vi "Reset.vi"(8 "error in (no error)":errorcluster, 9 "Mask":u64=16 format="x%x (b%b)", 10 "Set decimation":bool=TRUE, 11 "RP Instrument in":refnum<class "RP Instrument.lvclass">) -> (0 "error out":errorcluster, 3 "RP Instrument out":refnum<class "RP Instrument.lvclass">)   [LabVIEW 2024, in "RP Instrument.lvclass"]
uses:
  RP Instrument.lvclass
  RP Command.ctl
  RP Instrument.lvclass/RP Instrument.ctl
  RP Communicator/RP Communicator.lvclass
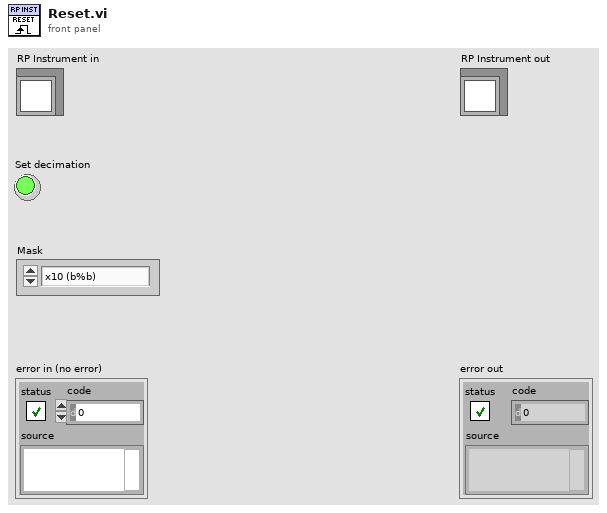
[diagram p1: front panel]
types:
  T1 = typedef "RP Command.ctl" = enum16{"Reset", "Read IDN", "Stop server", "Get status", "Get temperature", "Connect client", "Arm", "Software trigger", "Get whole buffer", "Get chunk", "System call", "Get config", "Set config", "Recieve data", "Recieve Calibartion", "Transmit data"}
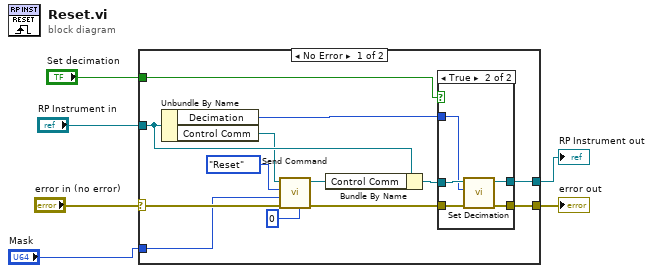
[diagram p0: block diagram]
diagram:
  n1 = case shown="No Error" "error in (no error)" {
    selector: "error in (no error)" -> [w15 w28]
    tunnel: [w13 w28] -> w5
    tunnel: [w11 w27] -> w3
    tunnel: "RP Instrument in" -> [w18 w27]
    tunnel: "Set decimation" -> [w10 _]
    tunnel: "Mask" -> [w7 _]
    frame No Error {
      n2 = Unbundle By Name(w18) -> ("Decimation"=w9:u32, "Control Comm"=w16:refnum<class "RP Communicator.lvclass">)
      n3 = call-dynamic "Send Command.vi"("bytes to read"=0, "error in (no error)"=w15, "Command payload"=w7, "Command number"=RP_Command."Reset", "RP Communicator in"=w16) -> ("error out"=w14:errorcluster, "RP Communicator out"=w17:refnum<class "RP Communicator.lvclass">)  [unwired: 4 in, 1 out]
      n4 = Bundle By Name(cluster=w18, "Control Comm"=w17) -> (w12:refnum<class "RP Instrument.lvclass">)
      n5 = case shown="True" w10 {
        tunnel: w14 -> [w20 w26]
        tunnel: [w20 w25] -> w13
        tunnel: w12 -> [w21 w24]
        tunnel: [w21 w23] -> w11
        tunnel: w9 -> [_ w22]
        frame False {
        }
        frame True {
          n6 = call-dynamic "Set Decimation.vi"("error in (no error)"=w26, "Decimation"=w22, "RP Instrument in"=w24) -> ("error out"=w25:errorcluster, "RP Instrument out"=w23:refnum<class "RP Instrument.lvclass">)  [unwired: 7 in]
        }
      }
    }
    frame Error {
    }
  }
  "error out" <- w5
  "RP Instrument out" <- w3
